vi "Cannon Sensors Update.vi"(1 "Cannon Information":T1) -> (0 "Cannon Information out":T1)   [LabVIEW 2012]
uses:
  BotStatus.vi
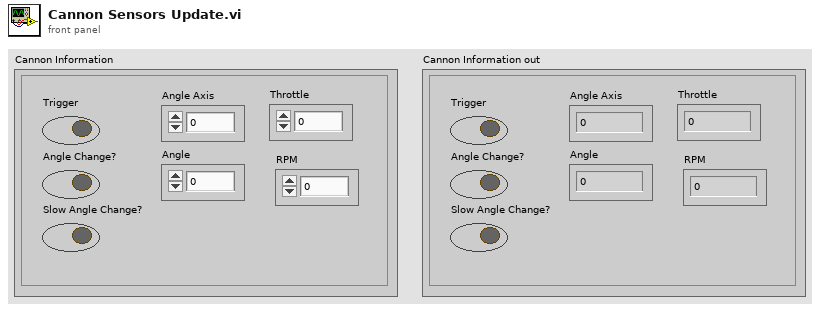
[diagram p1: front panel]
types:
  T1 = cluster{"RPM":dbl, "Trigger":bool, "Angle Axis":dbl, "Angle":dbl, "Throttle":dbl, "Slow Angle Change?":bool, "Angle Change?":bool}
  T2 = typedef "WPI_AnalogChannelDevRef.ctl" = cluster{"DevStatus":errorcluster, "Analog Module":T3, "Analog Channel":T4}
  T3 = typedef "FPGA_TypedefAnalogModule.ctl" = enum16{"Analog Module 1", "Analog Module 2"}
  T4 = typedef "FPGA_AIChannel.ctl" = enum8{"AI 1", "AI 2", "AI 3", "AI 4", "AI 5", "AI 6", "AI 7", "AI 8", "Invalid"}
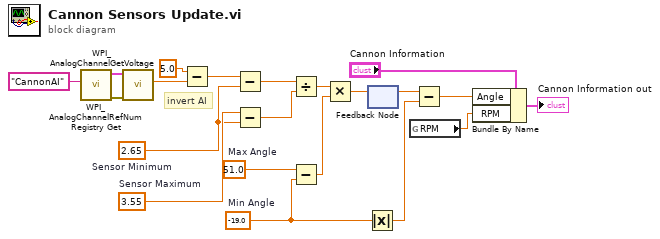
[diagram p0: block diagram]
diagram:
  w13 = 2.65  # Sensor Minimum
  w14 = 3.55  # Sensor Maximum
  w6 = 51.0  # Max Angle
  w5 = -19.0  # Min Angle
  # "invert AI"
  n1 = call <vilib>:"WPI_AnalogChannelRefNum Registry Get.vi"("refnum name"="CannonAI") -> ("error out"=w19:errorcluster, "AIDeviceRef"=w20:T2)  [unwired: 9 in]
  n2 = call <vilib>:"WPI_AnalogChannelGetVoltage.vi"("error in (no error)"=w19, "AIDeviceRef"=w20) -> ("Voltage"=w9:dbl)  [unwired: 7 in, 2 out]
  n3 = Subtract(x=5.0, y=w9) -> (x-y=w8:dbl)
  n4 = Subtract(x=w8, y=w13) -> (x-y=w11:dbl)
  n5 = Subtract(x=w14, y=w13) -> (x-y=w12:dbl)
  n6 = Divide(x=w11, y=w12) -> (x/y=w17:dbl)
  n7 = Subtract(x=w6, y=w5) -> (x-y=w18:dbl)
  n8 = Multiply(x=w17, y=w18) -> (x*y=w16:dbl)
  n9 = Absolute Value(x=w5) -> (abs(x)=w7:dbl)
  n10 = feedback #1() -> (w15:dbl)  [unwired: 1 in]
  n11 = feedback-in #1(w16) -> ()
  n12 = global read "BotStatus.vi" "RPM"() -> (w3:dbl)
  n13 = Subtract(x=w15, y=w7) -> (x-y=w4:dbl)
  n14 = Bundle By Name(cluster="Cannon Information", "Angle"=w4, "RPM"=w3) -> (→"Cannon Information out":T1)
